vi "Run Filter.vi"(8 "error in (no error)":errorcluster, 10 "resource entries in":T1[](array[typedef]) {"FPGA CD Ref" format="%.0x"; "reserver" format="%.0x"}, 11 "Reserver Filter in":refnum<class "Reserver Filter.lvclass">) -> (0 "error out":errorcluster, 2 "resource entries out":T1[](array[typedef]) {"FPGA CD Ref" format="%.0x"; "reserver" format="%.0x"})   [LabVIEW 2016, in "FPGA Resource Manager System Defintion.lvlib" / "Reserver Filter.lvclass"]
uses:
  Reserver Filter.lvclass
  resource info.ctl
  <vilib>/NI Veristand/Custom Device API/Custom Device Item Ref.ctl
  Reserver Filter.lvclass/Reserver Filter.ctl
  <vilib>/NI Veristand/Custom Device API/Custom Device API.lvlib
  FPGA Resource Manager System Defintion.lvlib
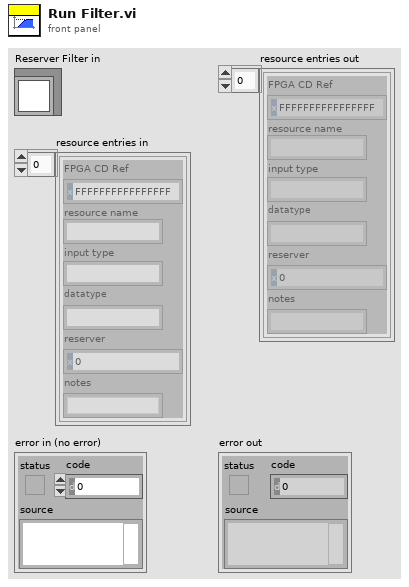
[diagram p1: front panel]
types:
  T1 = typedef "FPGA Resource Manager System Defintion.lvlib/resource info.ctl" = cluster{"FPGA CD Ref":T2, "resource name":string, "input type":string, "datatype":string, "reserver":T2, "notes":string}
  T2 = typedef "Custom Device API.lvlib/Custom Device Item Ref.ctl" = u64
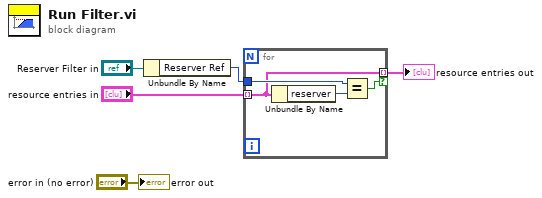
[diagram p0: block diagram]
diagram:
  n1 = Unbundle By Name("Reserver Filter in") -> ("Reserver Ref"=w3:T2)
  n2 = for {
    tunnel: w3 -> [w9]
    tunnel: "resource entries in" -> [w7] mode=indexing
    tunnel: [w7] -> w1 mode=indexing if=w6
    n3 = Unbundle By Name(w7) -> ("reserver"=w8:T2)
    n4 = Equal?(x=w9, y=w8) -> (x = y?=w6:bool)
  }
  "resource entries out" <- w1
  "error out" <- "error in (no error)"
